vi "Spectral Shape.vi"(4 "cutoff":dbl, 5 "Waveform":waveform(dbl), 6 "PSD[1]":dbl[](array[numeric]), 7 "PSD[0]":dbl[](array[numeric])) -> (0 "Zero Crossing":dbl, 1 "Spectral Rolloff":dbl, 2 "Spectral Flux":dbl, 3 "Spectral Centroid":dbl)   [LabVIEW 2013]
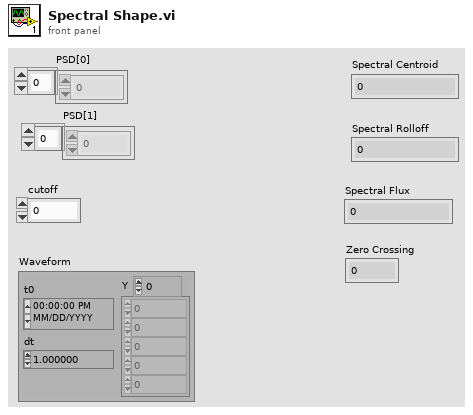
[diagram p1: front panel]
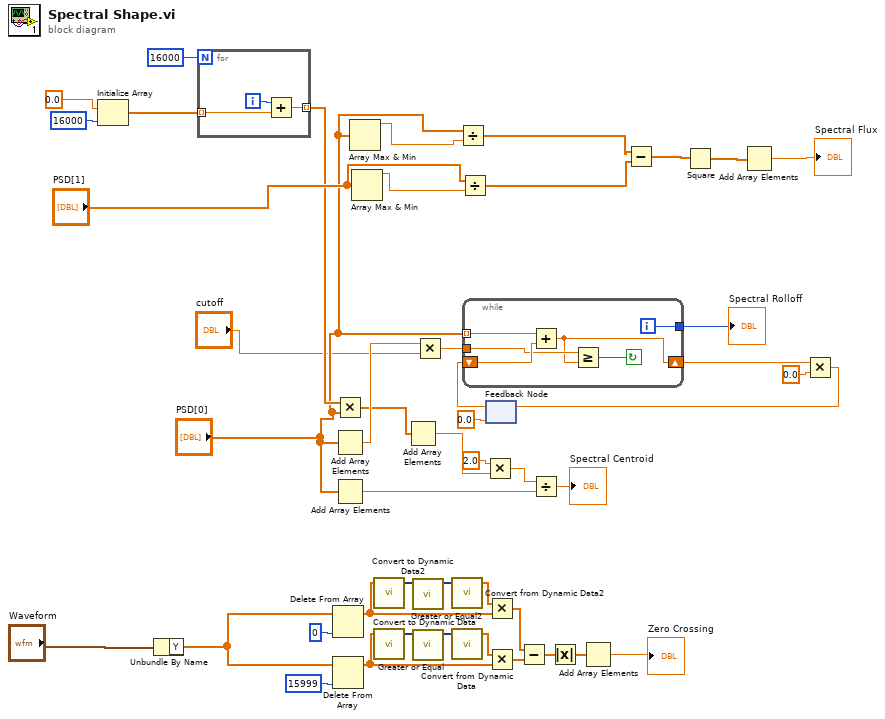
[diagram p0: block diagram]
diagram:
  n1 = Initialize Array(0.0 ("element"), 16000 ("dimension size")) -> (w30:dbl[])
  n2 = Unbundle By Name("Waveform") -> ("Y"=w3:dbl[])
  n3 = for {
    N: 16000 -> [_]
    tunnel: w30 -> [w49] mode=indexing
    tunnel: [w48] -> w21 mode=indexing
    i -> [w47]
    n4 = Add(x=w47, y=w49) -> (x+y=w48:dbl)
  }
  n5 = Delete From Array(array=w3, index=0) -> (array with subset deleted=w7:dbl[])  [unwired: 1 in, 1 out]
  n6 = Delete From Array(array=w3, index=15999) -> (array with subset deleted=w14:dbl[])  [unwired: 1 in, 1 out]
  n7 = Multiply(x=w21, y="PSD[0]") -> (x*y=w20:dbl[])
  n8 = Add Array Elements(numeric array="PSD[0]") -> (sum=w41:dbl)
  n9 = Add Array Elements(numeric array="PSD[0]") -> (sum=w42:dbl)
  n10 = Array Max & Min(array="PSD[0]") -> (max value=w26:dbl)  [unwired: 3 out]
  n11 = Array Max & Min(array="PSD[1]") -> (max value=w24:dbl)  [unwired: 3 out]
  n12 = call "Convert to Dynamic Data2"("Array"=w7) -> ("Dynamic Data Type"=w6:dynamicdata)  [unwired: 3 in]
  n13 = call "Convert to Dynamic Data"("Array"=w14) -> ("Dynamic Data Type"=w8:dynamicdata)  [unwired: 3 in]
  n14 = Add Array Elements(numeric array=w20) -> (sum=w45:dbl)
  n15 = call "Greater or Equal2"("Operand 1"=w6) -> ("Result"=w5:dynamicdata)  [unwired: 9 in, 1 out]
  n16 = call "Greater or Equal"("Operand 1"=w8) -> ("Result"=w11:dynamicdata)  [unwired: 9 in, 1 out]
  n17 = Multiply(x=w41, y="cutoff") -> (x*y=w38:dbl)
  n18 = call "Convert from Dynamic Data2"("Dynamic Data Type"=w5) -> ("Array"=w4:dbl[])  [unwired: 3 in]
  n19 = call "Convert from Dynamic Data"("Dynamic Data Type"=w11) -> ("Array"=w10:dbl[])  [unwired: 3 in]
  n20 = Divide(x="PSD[0]", y=w26) -> (x/y=w25:dbl[])
  n21 = Divide(x="PSD[1]", y=w24) -> (x/y=w23:dbl[])
  n22 = Multiply(x=2.0, y=w45) -> (x*y=w46:dbl)
  n23 = feedback #1(0.0) -> (w40:dbl)
  n24 = while {
    shift-right: [w50] -> w36
    shift-left: w40 -> [w55]
    tunnel: "PSD[0]" -> [w54] mode=indexing
    tunnel: [w53] -> w39
    tunnel: w38 -> [w51]
    i -> [w53]
    stop <- w52 continue-if-true
    n25 = Add(x=w54, y=w55) -> (x+y=w50:dbl)
    n26 = Greater Or Equal?(x=w51, y=w50) -> (x >= y?=w52:bool)
  }
  "Spectral Rolloff" <- w39
  n27 = Multiply(x=w4, y=w7) -> (x*y=w13:dbl[])
  n28 = Multiply(x=w10, y=w14) -> (x*y=w12:dbl[])
  n29 = Subtract(x=w13, y=w12) -> (x-y=w15:dbl[])
  n30 = Divide(x=w46, y=w42) -> (x/y=→"Spectral Centroid":dbl)
  n31 = Absolute Value(x=w15) -> (abs(x)=w9:dbl[])
  n32 = Add Array Elements(numeric array=w9) -> (sum=→"Zero Crossing":dbl)
  n33 = Subtract(x=w25, y=w23) -> (x-y=w29:dbl[])
  n34 = Square(x=w29) -> (x^2=w28:dbl[])
  n35 = Add Array Elements(numeric array=w28) -> (sum=→"Spectral Flux":dbl)
  n36 = Multiply(x=w36, y=0.0) -> (x*y=w34:dbl)
  n37 = feedback-in #1(w34) -> ()
